vi "ma_piture.vi"(8 "Error":errorcluster, 11 "KNR in":T2) -> (0 "error out":errorcluster, 1 "Number of Matches (Shape Detection 1)":i32, 2 "Circles (Shape Detection 1)":T4(array[cluster]) {"Position"."Y" format="%.2f"; "Position"."X" format="%.2f"}, 3 "KNR out":T2, 5 "Image Out":T1)   [LabVIEW 2013]
uses:
  <userlib>/KNR OS 3.0 LabVIEW Toolkit/Type Definition/KNR3 Reference.ctl
  <userlib>/_FPGA Interface Advanced Tools/FPGA Interface Base/FPGA Interface Base.lvclass
  <userlib>/KNR OS 3.0 LabVIEW Toolkit/Type Definition/Resource.ctl
  <vilib>/vision/Image Controls.llb/IMAQ Image.ctl
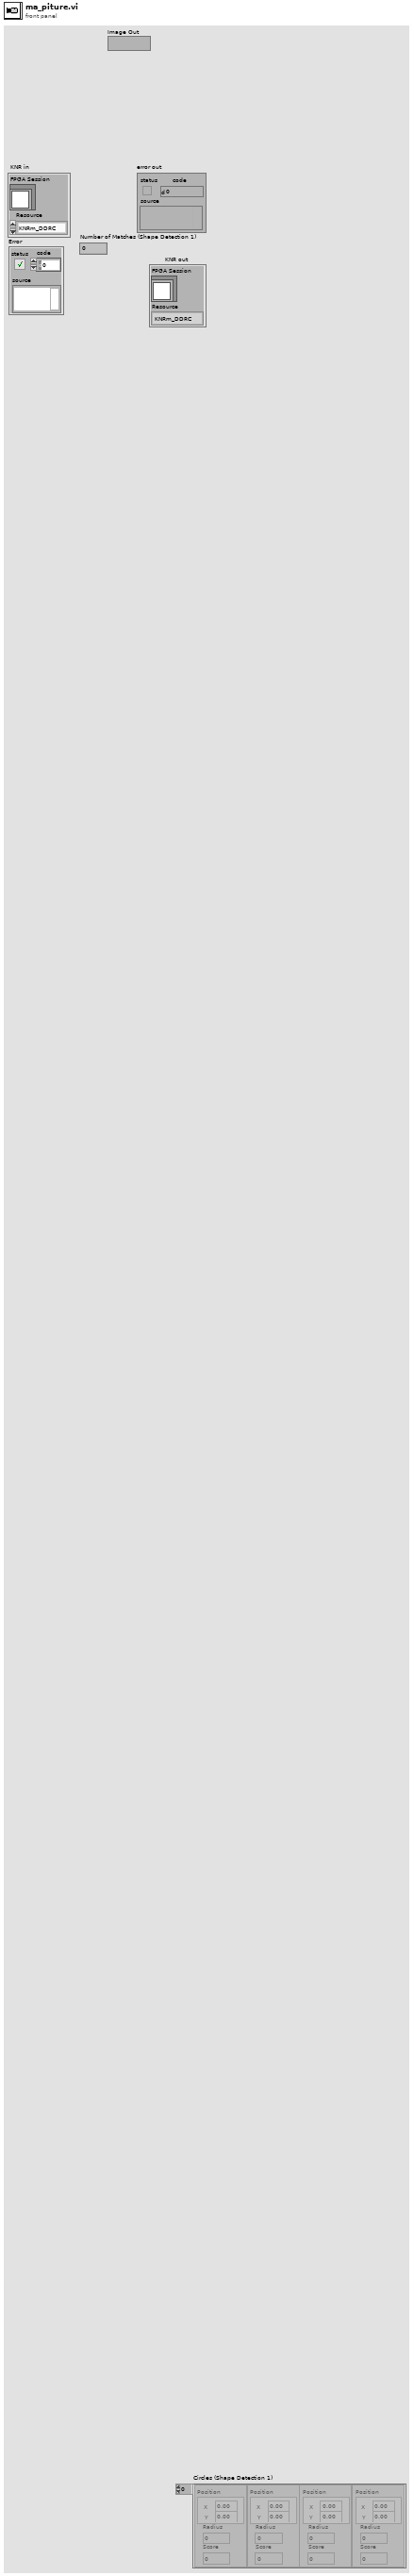
[diagram p1: front panel]
types:
  T1 = typedef "IMAQ Image.ctl" = refnum<image>
  T2 = typedef "KNR3 Reference.ctl" = cluster{"FPGA Session":refnum<class "FPGA Interface Base.lvclass">, "Resource":T3}
  T3 = typedef "Resource.ctl" = enum16{"KNRm_DDRC", "KNRm_DDDD", "KNRm_DDDR", "KNRm_DDDC", "KNR"}
  T4 = cluster{"Position":cluster{"X":sgl, "Y":sgl}, "Radius":dbl, "Score":dbl}[]
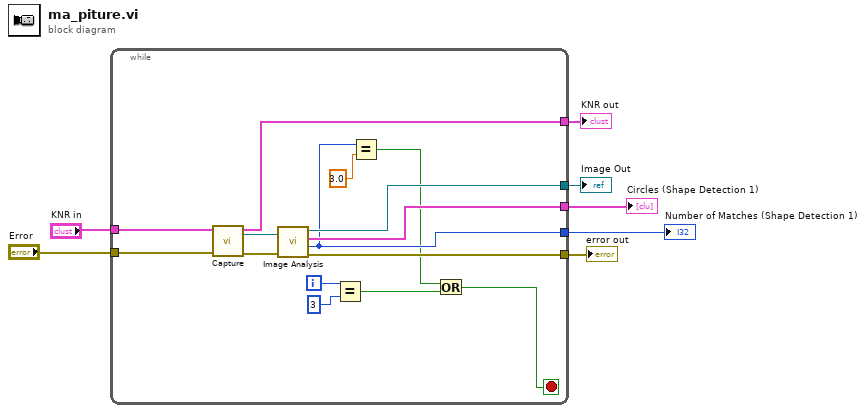
[diagram p0: block diagram]
diagram:
  n1 = while {
    tunnel: "KNR in" -> [w20]
    tunnel: "Error" -> [w19]
    tunnel: [w18] -> w5
    tunnel: [w17] -> w4
    tunnel: [w16] -> w3
    tunnel: [w13] -> w2
    tunnel: [w8] -> w1
    i -> [w15]
    stop <- w9 stop-if-true
    n2 = call "Capture.vi"("Error"=w19, "KNR in"=w20) -> ("error out"=w21:errorcluster, "Image Out"=w22:T1, "KNR out"=w8:T2)  [unwired: 7 in]
    n3 = call "Image Analysis.vi"("Image In"=w22, "error in"=w21) -> ("Image Out"=w18:T1, "Circles (Shape Detection 1)"=w17:T4, "Number of Matches (Shape Detection 1)"=w13:i32, "error out"=w16:errorcluster)
    n4 = Equal?(x=w15, y=3) -> (x = y?=w10:bool)
    n5 = Equal?(x=w13, y=3.0) -> (x = y?=w11:bool)
    n6 = Or(x=w11, y=w10) -> (x .or. y?=w9:bool)
  }
  "Circles (Shape Detection 1)" <- w4
  "error out" <- w3
  "Number of Matches (Shape Detection 1)" <- w2
  "KNR out" <- w1
  "Image Out" <- w5
